vi "Network Endpoint A.vi"() -> ()   [LabVIEW 2020]
uses:
  Communication/IP_Communication/typedefs/General Settings.ctl
  Communication/IP_Communication/typedefs/Endpoint Tag.ctl
  Communication VIs/Network/Network Settings.ctl
  Communication VIs/Network/Network.lvlib
  Communication/IP_Communication/IP_Communication.lvclass
panel:
  in  "Network Settings":T1={"Peer IP Address"="localhost"}
  in  "General Settings":T2={"Connection Name"="Network_Test", "Endpoint Tag"=enum."A"}
  in  "Stop VI":bool
  in  "Send Command":bool
  in  "Command ID":u16
  out "Command Rx":T4
  out "Timeout?":bool
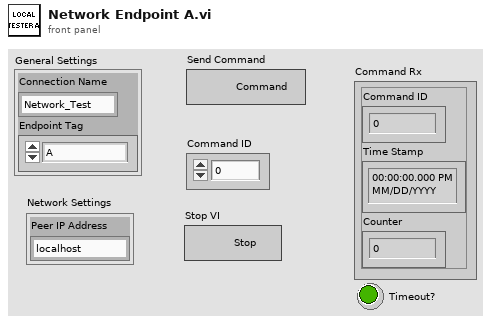
[diagram p1: front panel]
types:
  T1 = typedef "Communication VIs.lvlib/Network.lvlib/Network Settings.ctl" = cluster{"Peer IP Address":string}
  T2 = typedef "Communication Classes.lvlib/IP_Communication.lvclass/General Settings.ctl" = cluster{"Connection Name":string, "Endpoint Tag":T3}
  T3 = typedef "Communication Classes.lvlib/IP_Communication.lvclass/Endpoint Tag.ctl" = enum8{"A", "B"}
  T4 = cluster{"Command ID":u16, "Time Stamp":timestamp, "Counter":u16}
  T5 = cluster{"Command Out":cluster{"Command ID":u16, "Time Stamp":timestamp, "Counter":u16}, " Timeout?":bool}
  T6 = typedef "Communication VIs.lvlib/Network.lvlib/Network Streams.ctl" = cluster{"Tx_Endpoint":refnum<k21>, "Rx_Endpoint":refnum<k21>}
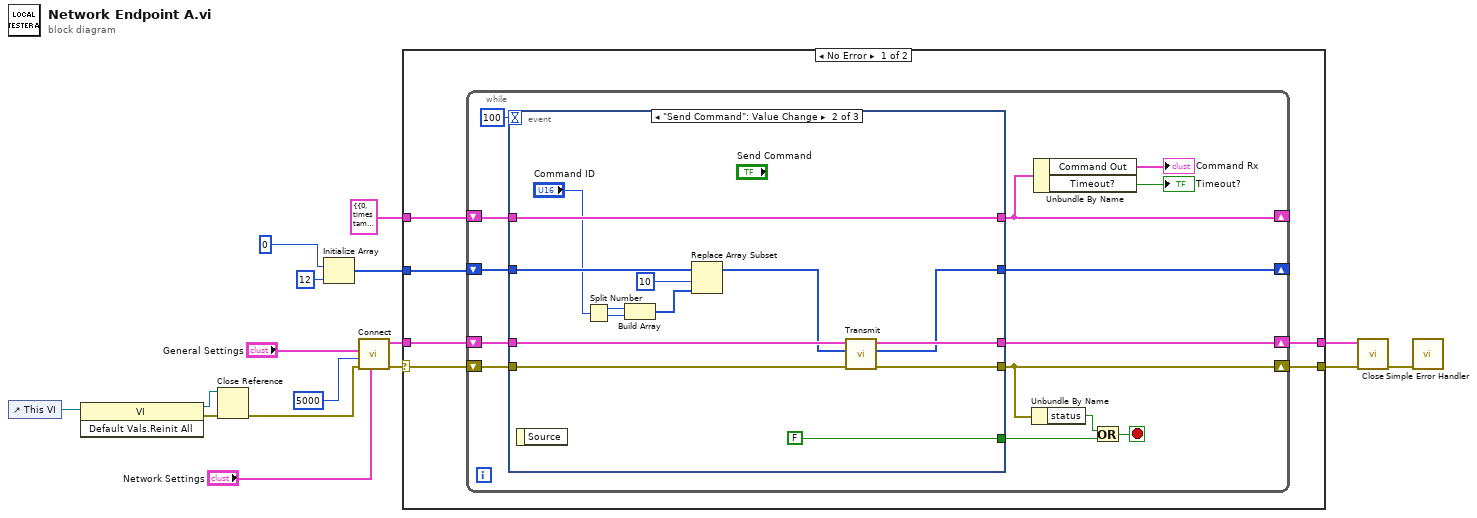
[diagram p0: block diagram]
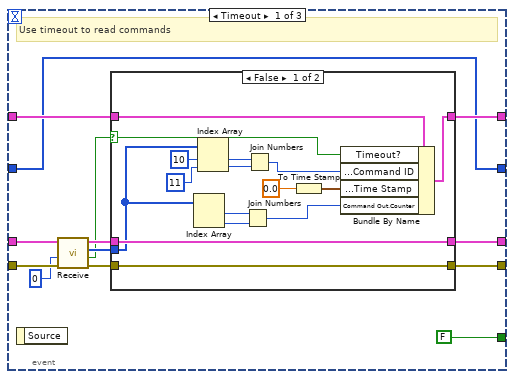
[diagram p2: hidden frame]
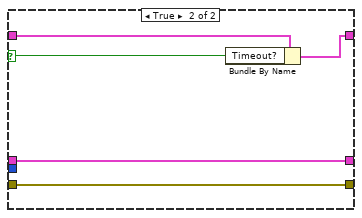
[diagram p3: hidden frame]
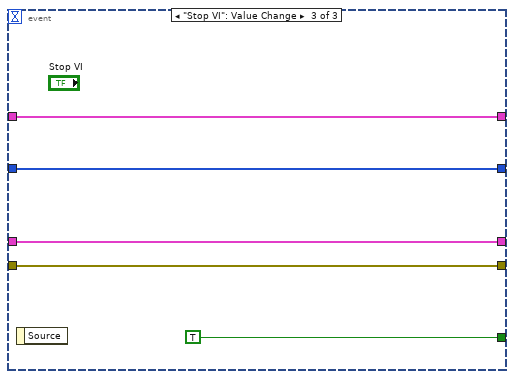
[diagram p4: hidden frame]
diagram:
  n1 = control-ref of="This VI"() -> (w13:refnum<vi>)
  n2 = invoke class="VI" method="Default Vals.Reinit All"(reference=w13) -> (reference out=w11:refnum<vi>, error out=w12:errorcluster)  [unwired: 2 in, 1 out]
  n3 = Close Reference(reference=w11, error in (no error)=w12) -> (error out=w6:errorcluster)
  n4 = Initialize Array(u8 0, 12 ("dimension size")) -> (w3:u8[])
  n5 = call "Connect.vi"("Network Settings"="Network Settings", "error in (no error)"=w6, "timeout in ms (10000)"=5000 ("Timeout"), "General Settings"="General Settings") -> ("error out"=w15:errorcluster, "Network_Streams out"=w14:T6)  [unwired: 6 in]
  n6 = case shown="No Error" w15 {
    selector: w15 -> [w22 w91]
    tunnel: [w19 w91] -> w9
    tunnel: [w18 w90] -> w2
    tunnel: w14 -> [w21 w90]
    tunnel: T5 {"Command Out"={"Command ID"=0, "Time Stamp"=timestamp(0 s since 1904-01-01), "Counter"=0}, " Timeout?"=FALSE} -> [w20 _]
    tunnel: w3 -> [w17 _]
    frame No Error {
      n7 = while {
        shift-right: [w31] -> _
        shift-left: w20 -> [w35]
        shift-right: [w32] -> w18
        shift-left: w21 -> [w34]
        shift-right: [w28] -> w19
        shift-left: w22 -> [w33]
        shift-right: [w23] -> _
        shift-left: w17 -> [w24]
        stop <- w27 stop-if-true
        n8 = event shown="[1] \"Send Command\": Value Change" {
          selector: _ -> [_ _ _]
          dyn-events: _ -> [_ _ _]
          timeout: 100 -> [_ _ _]
          tunnel: w35 -> [w41 w84 w89]
          tunnel: [w40 w84 w89] -> w31
          tunnel: w34 -> [w38 w81 w88]
          tunnel: w33 -> [w48 w73 w87]
          tunnel: [w46 w83 w87] -> w28
          tunnel: [w37 w72 w88] -> w32
          tunnel: [FALSE FALSE TRUE] -> w25
          tunnel: w24 -> [w39 w76 w85]
          tunnel: [w39 w71 w85] -> w23
          event Timeout {
            # "Use timeout to read commands"
            n9 = event-data() -> ()  [unwired: 1 in, 1 out]
            n10 = call "Receive.vi"("error in (no error)"=w48, "timeout in ms (0)"=0 ("timeout in ms (-1)"), "Network_Streams in"=w38) -> ("error out"=w49:errorcluster, "Timeout?"=w42:bool, "Packet Data"=w44:u8[], "Network_Streams out"=w47:T6)  [unwired: 5 in]
            n11 = case shown="False" w42 {
              selector: w42 -> [w63 w67]
              tunnel: w49 -> [w60 w69]
              tunnel: w47 -> [w62 w70]
              tunnel: [w60 w69] -> w46
              tunnel: [w62 w70] -> w37
              tunnel: w44 -> [w50 _]
              tunnel: w41 -> [w65 w68]
              tunnel: [w64 w66] -> w40
              frame False {
                n12 = Index Array(array=w50) -> (element #1=w58:u8, element #2=w57:u8)  [unwired: 2 in]
                n13 = Index Array(array=w50, index #1=10 ("index"), index #2=11 ("index")) -> (element #1=w54:u8, element #2=w55:u8)
                n14 = Join Numbers(hi=w58, lo=w57) -> ((hi.lo)=w56:u16)
                n15 = Join Numbers(hi=w54, lo=w55) -> ((hi.lo)=w51:u16)
                n16 = To Time Stamp(1:0.0 ("number")) -> (0:w61:timestamp)
                n17 = Bundle By Name(cluster=w65, "Timeout?"=w63, "Command Out.Command ID"=w51, "Command Out.Time Stamp"=w61, "Command Out.Counter"=w56) -> (w64:T5)
              }
              frame True {
                n18 = Bundle By Name(cluster=w68, "Timeout?"=w67) -> (w66:T5)
              }
            }
          }
          event "Send Command": Value Change {
            n19 = event-data() -> ()  [unwired: 1 in, 1 out]
            n20 = Split Number(x="Command ID") -> (hi(x)=w78:u8, lo(x)=w79:u8)
            n21 = Build Array(w78, w79) -> (w80:u8[])
            n22 = Replace Array Subset "Replace Array Subset"(array=w76, new element=w80, index=10) -> (w74:u8[])
            n23 = call "Transmit.vi"("error in (no error)"=w73, "Packet Data"=w74, "Network_Streams in"=w81) -> ("error out"=w83:errorcluster, "Packet Data Sent"=w71:u8[], "Network_Streams out"=w72:T6)  [unwired: 5 in, 1 out]
          }
          event "Stop VI": Value Change {
            n24 = event-data() -> ()  [unwired: 1 in, 1 out]
          }
        }
        n25 = Unbundle By Name(w28) -> ("status"=w26:bool)
        n26 = Unbundle By Name(w31) -> ("Command Out"=→"Command Rx":T4, "Timeout?"=→"Timeout?":bool)
        n27 = Or(x=w26, y=w25) -> (x .or. y?=w27:bool)
      }
    }
    frame Error {
    }
  }
  n28 = call "Close.vi"("error in (no error)"=w9, "Network_Streams in"=w2) -> ("error out"=w16:errorcluster)  [unwired: 9 in]
  n29 = call <vilib>:"Simple Error Handler.vi"("error in (no error)"=w16) -> ()  [unwired: 4 in, 5 out]
